vi "measure.vi"(8 "error in":errorcluster, 10 "pin map id":string, 11 "measurement configuration":cluster{"Boolean":bool}) -> (0 "error out":errorcluster, 3 "measurement results":cluster{"Boolean":bool})   [LabVIEW 2021, in "Measurement Client Template.lvlib"]
uses:
  Measurement Client Template.lvlib
  <vilib>/gRPC/Generated APIs/ni/measurementlink/measurement/v2/Measurement Service Client/RPC Messages/ni_measurementlink_measurement_v2_MeasureRequest.ctl
  <vilib>/gRPC/Generated APIs/ni/measurementlink/measurement/v2/Measurement Service Client/RPC Messages/google_protobuf_Any.ctl
  <vilib>/gRPC/Generated APIs/ni/measurementlink/measurement/v2/Measurement Service Client/RPC Messages/ni_measurementlink_PinMapContext.ctl
  <vilib>/gRPC/Generated APIs/ni/measurementlink/discovery/v1/RPC Messages/ni_measurementlink_discovery_v1_ResolveServiceRequest.ctl
  17d0f289-ea27-4c60-b0eb-587fd1b50e65.vi
  483b5dc2-6359-43fd-90c2-457bf83eb633.vi
  <vilib>/gRPC/LabVIEW gRPC Library/Server API/Translate Protobuf Error.vi
  <vilib>/AdvancedString/1D String Array to Delimited String.vi
  <vilib>/gRPC/LabVIEW gRPC Library/Server API/Server/Get Server DLL Path.vi
  <vilib>/gRPC/Generated APIs/ni/measurementlink/measurement/v2/Measurement Service Client/Measurement Service Client.lvlib
  <vilib>/gRPC/LabVIEW gRPC Library/grpc-lvsupport-release.lvlib
  <vilib>/gRPC/Generated APIs/ni/measurementlink/discovery/v1/ni.measurementlink.discovery.v1.api.lvlib
  <vilib>/Plug-In SDKs/Clients/Discovery V1/NI Discovery V1 Client.lvlib
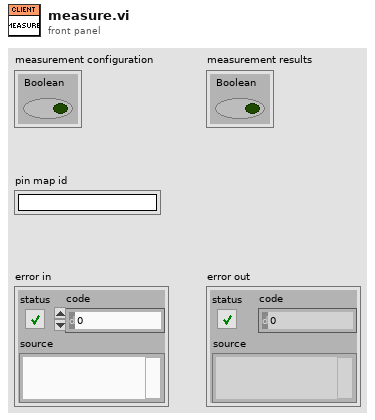
[diagram p1: front panel]
types:
  T1 = typedef "ni.measurementlink.discovery.v1.api.lvlib/ni_measurementlink_discovery_v1_ResolveServiceRequest.ctl" = cluster{"provided_interface":string, "service_class":string}
  T2 = typedef "ni.measurementlink.measurement.v2.api.lvlib/Measurement Service Client.lvlib/ni_measurementlink_measurement_v2_MeasureRequest.ctl" = cluster{"configuration_parameters":T3, "pin_map_context":T4}
  T3 = typedef "ni.measurementlink.measurement.v2.api.lvlib/Measurement Service Client.lvlib/google_protobuf_Any.ctl" = cluster{"type_url":string, "value":u8[]}
  T4 = typedef "ni.measurementlink.measurement.v2.api.lvlib/Measurement Service Client.lvlib/ni_measurementlink_PinMapContext.ctl" = cluster{"pin_map_id":string, "sites":i32[]}
  T5 = typedef "grpc-lvsupport-release.lvlib/grpcId.ctl" = u64
  T6 = typedef "ni.measurementlink.discovery.v1.api.lvlib/ni_measurementlink_discovery_v1_ServiceLocation.ctl" = cluster{"location":string, "insecure_port":string, "ssl_authenticated_port":string}
  T7 = typedef "grpc-lvsupport-release.lvlib/Enum Metadata.ctl" = cluster{"Version":i32, "Name":string, "Type Url":string, "Enum Values":string, "Allow Alias":bool}
  T8 = typedef "grpc-lvsupport-release.lvlib/Message Metadata.ctl" = cluster{"Version":i32, "Name":string, "Type Url":string, "Elements":T9[], "Has Oneof":bool}
  T9 = typedef "grpc-lvsupport-release.lvlib/Message Element Metadata.ctl" = cluster{"Field Name":string, "Embedded Message Name":string, "Protobuf Index":i32, "MessageElementType":T10, "Repeated":bool, "Is in Oneof":bool, "Oneof Container Name":string}
  T10 = typedef "grpc-lvsupport-release.lvlib/Message Element Type.ctl" = enum32{"Int32Value", "FloatValue", "DoubleValue", "BoolValue", "StringValue", "MessageValue", "Int64Value", "UInt32Value", "UInt64Value", "EnumValue", "Bytes", "Fixed64", "Fixed32", "SFixed64", "SFixed32", "SInt64", "SInt32"}
  T11 = typedef "grpc-lvsupport-release.lvlib/Any.ctl" = cluster{"Type Url":string, "Bytes":u8[]}
  T12 = typedef "ni.measurementlink.measurement.v2.api.lvlib/Measurement Service Client.lvlib/ni_measurementlink_measurement_v2_MeasureResponse.ctl" = cluster{"outputs":T3}
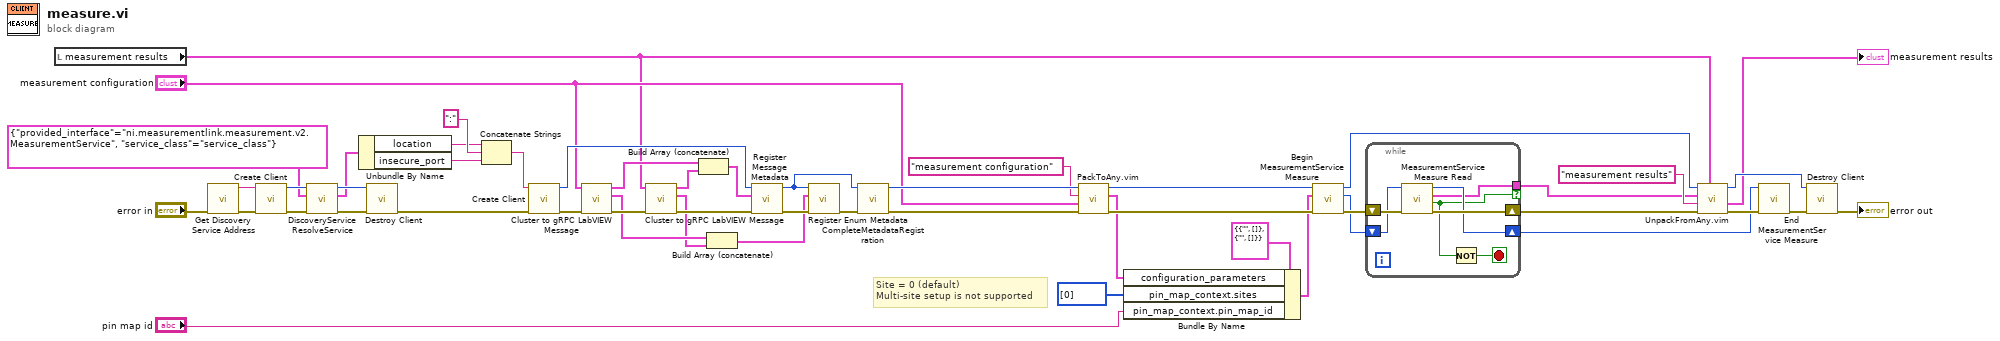
[diagram p0: block diagram]
diagram:
  # "Site = 0 (default)\nMulti-site setup is not supported"
  n1 = local read "measurement results"() -> (w29:cluster{"Boolean":bool})
  n2 = call <vilib>:"Get Discovery Service Address.vi"("error in"="error in") -> ("error out"=w7:errorcluster, "address"=w6:string)  [unwired: 9 in]
  n3 = call <vilib>:"Create Client.vi"("error in"=w7, "address"=w6) -> ("error out"=w10:errorcluster, "gRPC ID Out"=w9:T5)  [unwired: 8 in]
  n4 = call <vilib>:"DiscoveryService ResolveService.vi"("error in"=w10, "Request Data"=T1 {"provided_interface"="ni.measurementlink.measurement.v2.MeasurementService", "service_class"="service_class"} ("resolve service request data"), "gRPC ID"=w9) -> ("error out"=w13:errorcluster, "Response Data"=w11:T6, "gRPC ID out"=w12:T5)  [unwired: 6 in]
  n5 = Unbundle By Name(w11) -> ("location"=w48:string, "insecure_port"=w49:string)
  n6 = call <vilib>:"Destroy Client.vi"("error in"=w13, "gRPC ID"=w12) -> ("error out"=w14:errorcluster)  [unwired: 9 in]
  n7 = Concatenate Strings(w48, ":" ("string"), w49) -> (w50:string)
  n8 = call <vilib>:"Create Client.vi"("error in"=w14, "address"=w50) -> ("error out"=w46:errorcluster, "gRPC ID Out"=w39:T5)  [unwired: 8 in]
  n9 = call <vilib>:"Cluster to gRPC LabVIEW Message.vi"("error in"=w46, "Cluster"="measurement configuration") -> ("error out"=w47:errorcluster, "gRPC Enum Metadata out"=w16:T7[], "gRPC Message Metadata []"=w40:T8[])  [unwired: 7 in]
  n10 = call <vilib>:"Cluster to gRPC LabVIEW Message.vi"("error in"=w47, "Cluster"=w29) -> ("error out"=w43:errorcluster, "gRPC Enum Metadata out"=w15:T7[], "gRPC Message Metadata []"=w42:T8[])  [unwired: 7 in]
  n11 = Build Array (concatenate)(w40, w42) -> (w41:T8[])
  n12 = Build Array (concatenate)(w16, w15) -> (w17:T7[])
  n13 = call <vilib>:"Register Message Metadata.vi"("error in"=w43, "Messages"=w41, "gRPCid in"=w39) -> ("error out"=w19:errorcluster, "gRPCid out"=w2:T5)  [unwired: 7 in]
  n14 = call <vilib>:"Register Enum Metadata.vi"("error in"=w19, "Enum Metadata"=w17, "gRPCid in"=w2) -> ("error out"=w18:errorcluster)  [unwired: 7 in, 1 out]
  n15 = call <vilib>:"CompleteMetadataRegistration.vi"("error in"=w18, "gRPC ID in"=w2) -> ("error out"=w44:errorcluster, "gRPC ID Out"=w45:T5)  [unwired: 8 in]
  n16 = call "PackToAny.vim"("error in"=w44, "Data To Pack"="measurement configuration", "Message Type"="measurement configuration", "gRPCid in"=w45) -> ("error out"=w36:errorcluster, "Any"=w35:T11, "gRPCid out"=w20:u64)  [unwired: 5 in]
  n17 = Bundle By Name(cluster=T2 {"configuration_parameters"={"type_url"="", "value"=[]}, "pin_map_context"={"pin_map_id"="", "sites"=[]}} ("Request Data"), "configuration_parameters"=w35, "pin_map_context.sites"=i32[] [0], "pin_map_context.pin_map_id"="pin map id") -> (w34:T2)
  n18 = call <vilib>:"Begin MeasurementService Measure.vi"("error in"=w36, "Request Data"=w34, "gRPC ID"=w20) -> ("error out"=w33:errorcluster, "Call Id Out"=w26:T5, "gRPC ID out"=w24:T5)  [unwired: 6 in]
  n19 = while {
    shift-right: [w57] -> w32
    shift-left: w33 -> [w58]
    shift-right: [w55] -> w25
    shift-left: w26 -> [w56]
    tunnel: [w53] -> w1 if=w52
    stop <- w54 stop-if-true
    n20 = call <vilib>:"MeasurementService Measure Read.vi"("error in"=w58, "Call ID in"=w56) -> ("error out"=w57:errorcluster, "Success"=w52:bool, "Response Data"=w53:T12, "Call ID"=w55:T5)  [unwired: 6 in]
    n21 = Not(x=w52) -> (.not. x?=w54:bool)
  }
  n22 = call "UnpackFromAny.vim"("Data Type"=w29, "error in"=w32, "Message Type"="measurement results", "Any"=w1, "gRPCid in"=w24) -> ("error out"=w28:errorcluster, "Unpacked Value"=→"measurement results":cluster{"Boolean":bool}, "gRPCid out"=w23:u64)  [unwired: 4 in]
  n23 = call <vilib>:"End MeasurementService Measure.vi"("error in"=w28, "Call ID in"=w25) -> ("error out"=w27:errorcluster)  [unwired: 8 in, 1 out]
  n24 = call <vilib>:"Destroy Client.vi"("error in"=w27, "gRPC ID"=w23) -> ("error out"=→"error out":errorcluster)  [unwired: 9 in]
